vi "02Control.vi"(0 "Config equipo":T1, 1 "001":bool, 2 "010":bool, 3 "100":bool, 4 "000":bool) -> (5 "error out":errorcluster)   [LabVIEW 2010]
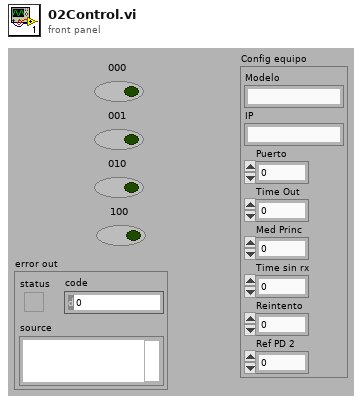
[diagram p1: front panel]
types:
  T1 = cluster{"Modelo":string, "IP":string, "Puerto":u16, "Time Out":u16, "Med Princ":u16, "Time sin rx":u16, "Reintento":u16, "Ref PD 2":u16}
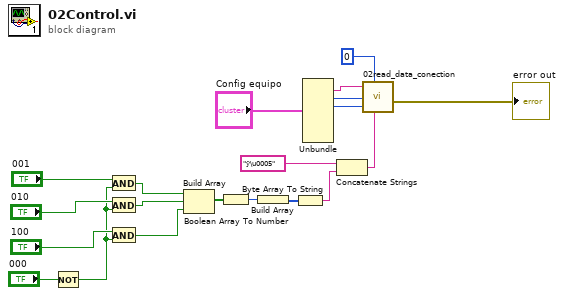
[diagram p0: block diagram]
diagram:
  n1 = Not(x="000") -> (.not. x?=w1:bool)
  n2 = And(x="001", y=w1) -> (x .and. y?=w7:bool)
  n3 = And(x="010", y=w1) -> (x .and. y?=w6:bool)
  n4 = And(x="100", y=w1) -> (x .and. y?=w5:bool)
  n5 = Build Array(w7, w6, w5) -> (w9:bool[])
  n6 = Boolean Array To Number(Boolean array=w9) -> (number=w18:u32)
  n7 = Build Array(w18) -> (w17:u32[])
  n8 = Byte Array To String(unsigned byte array=w17) -> (string=w16:string)
  n9 = Unbundle("Config equipo") -> ("IP"=w14:string, "Puerto"=w13:u16, "Time Out"=w12:u16)  [unwired: 5 out]
  n10 = Concatenate Strings("ÿ\u0005", w16) -> (w11:string)
  n11 = call "02read_data_conection.vi"("IP"=w14, "bytes to read"=u8 0, "Puerto"=w13, "Time Out"=w12, "string to write"=w11) -> ("error out"=→"error out":errorcluster)  [unwired: 1 out]
